vi "Edge Detection (zero encoder).vi"(2 "limitSwitch[]":bool[](array[boolean])) -> (0 "zeroEncoders":bool[](array[boolean]))   [LabVIEW 2019]
uses:
  swerveData.vi
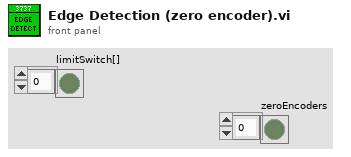
[diagram p1: front panel]
types:
  T1 = cluster{"[0]":bool, "[1]":bool, "[2]":bool, "[3]":bool, "[4]":bool, "[5]":bool, "[6]":bool, "[7]":bool, "[8]":bool}
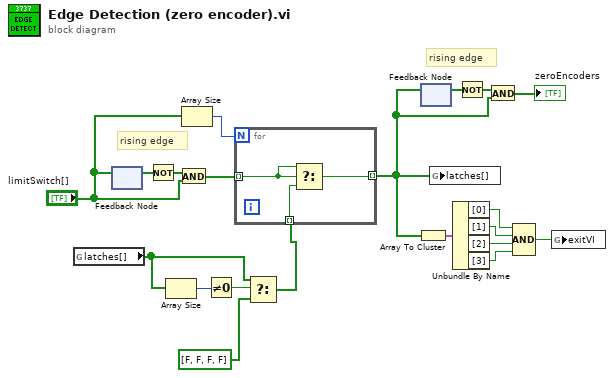
[diagram p0: block diagram]
diagram:
  # "rising edge"
  # "rising edge"
  n1 = global read "swerveData.vi" "latches[]"() -> (w3:bool[])
  n2 = feedback #1() -> (w19:bool[])  [unwired: 1 in]
  n3 = feedback-in #1("limitSwitch[]") -> ()
  n4 = Not(x=w19) -> (.not. x?=w20:bool[])
  n5 = Array Size(array=w3) -> (size(s)=w5:i32)
  n6 = And(x=w20, y="limitSwitch[]") -> (x .and. y?=w8:bool[])
  n7 = Array Size(array="limitSwitch[]") -> (size(s)=w7:i32)
  n8 = Not Equal To 0?(x=w5) -> (x != 0?=w4:bool)
  n9 = Select(t=w3, s=w4, f=bool[] [FALSE, FALSE, FALSE, FALSE] ("limitSwitch[]")) -> (s? t:f=w1:bool[])
  n10 = for {
    N: w7 -> [_]
    tunnel: w1 -> [w23] mode=indexing
    tunnel: [w22] -> w16 mode=indexing
    tunnel: w8 -> [w21] mode=indexing
    n11 = Select(t=w21, s=w21, f=w23) -> (s? t:f=w22:bool)
  }
  n12 = Array To Cluster(array=w16) -> (cluster=w14:T1)
  n13 = feedback #2() -> (w18:bool[])  [unwired: 1 in]
  n14 = feedback-in #2(w16) -> ()
  n15 = global write "swerveData.vi" "latches[]"(w16) -> ()
  n16 = Unbundle By Name(w14) -> ("[0]"=w13:bool, "[1]"=w10:bool, "[2]"=w11:bool, "[3]"=w12:bool)
  n17 = Not(x=w18) -> (.not. x?=w17:bool[])
  n18 = And(x=w17, y=w16) -> (x .and. y?=→"zeroEncoders":bool[])
  n19 = Compound Arithmetic op=AND(w13, w10, w11, w12) -> (w9:bool)
  n20 = global write "swerveData.vi" "exitVI"(w9) -> ()
